vi "ResetChips.vi"(8 "error in (no error)":errorcluster, 10 "LayerID":u32=65535 format="%x", 11 "connection ID":refnum<k5>) -> (0 "error out":errorcluster, 3 "connection ID out":refnum<k5>, 4 "Reset done":string)   [LabVIEW 2015, in "VIPM2.lvlib"]
uses:
  VIPM2.lvlib
panel:
  out "Ready to receive parameters":string
  # "RESET"
  # "Resets the chips of the indicated layer."
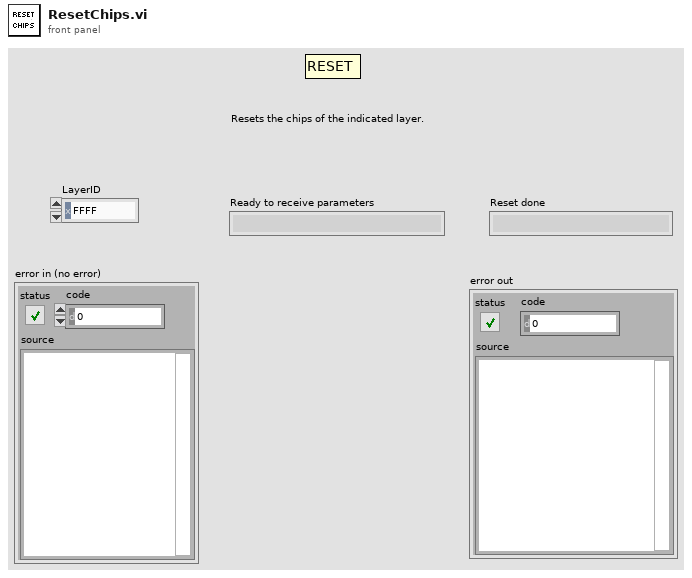
[diagram p1: front panel]
types:
  T1 = enum16{"Standard", "Buffered", "CRLF", "Immediate"}
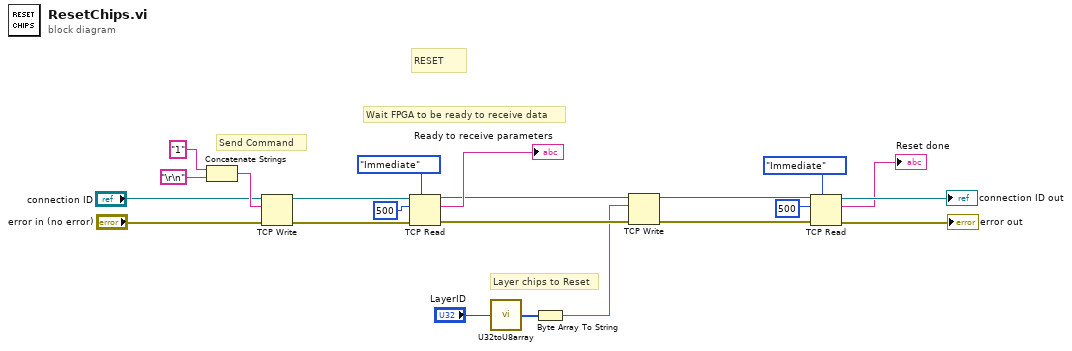
[diagram p0: block diagram]
diagram:
  # "Layer chips to Reset"
  # "Wait FPGA to be ready to receive data"
  # "Send Command"
  # "RESET"
  n1 = Concatenate Strings("1" ("string"), "\r\n") -> (w20:string)
  n2 = TCP Write(connection ID="connection ID", data in=w20, error in (no error)="error in (no error)") -> (connection ID out=w14:refnum<k5>, error out=w13:errorcluster)  [unwired: 1 in, 1 out]
  n3 = TCP Read(connection ID=w14, bytes to read=500, error in (no error)=w13, 7:T1."Immediate" ("mode (standard)")) -> (connection ID out=w10:refnum<k5>, data out=→"Ready to receive parameters":string, error out=w9:errorcluster)  [unwired: 1 in]
  n4 = call "U32toU8array.vi"("x"="LayerID") -> ("ArrayU8"=w11:u8[])
  n5 = Byte Array To String(unsigned byte array=w11) -> (string=w8:string)
  n6 = TCP Write(connection ID=w10, data in=w8, error in (no error)=w9) -> (connection ID out=w5:refnum<k5>, error out=w4:errorcluster)  [unwired: 1 in, 1 out]
  n7 = TCP Read(connection ID=w5, bytes to read=500, error in (no error)=w4, 7:T1."Immediate" ("mode (standard)")) -> (connection ID out=→"connection ID out":refnum<k5>, data out=→"Reset done":string, error out=→"error out":errorcluster)  [unwired: 1 in]
